vi "Errorbar1000.vi"   [LabVIEW 2013]
uses:
  <vilib>/Heliosphere Research LLC/Advanced Plotting Toolkit/Advanced Plotting Toolkit.lvlib
types:
  T1 = typedef "Advanced Plotting Toolkit.lvlib/PlotID.ctl" = i32
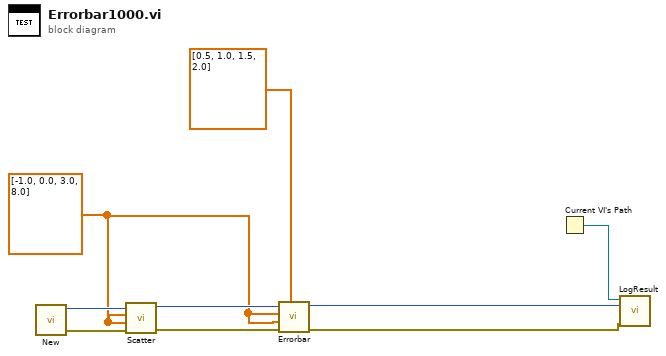
[diagram p0: block diagram]
diagram:
  w2 = dbl[] [-1.0, 0.0, 3.0, 8.0] ("X Data")
  n1 = call <vilib>:"New.vi"() -> ("error out"=w3:errorcluster, "Plot ID"=w6:T1)  [unwired: 10 in]
  n2 = call <vilib>:"Scatter.vi"("error in (no error)"=w3, "Y Data"=w2, "X Data"=w2, "Plot ID"=w6) -> ("error out"=w4:errorcluster, "Plot ID Out"=w5:T1)  [unwired: 6 in]
  n3 = call <vilib>:"Errorbar.vi"("X Errors"=dbl[] [0.5, 1.0, 1.5, 2.0], "error in (no error)"=w4, "Y Data"=w2, "X Data"=w2, "Plot ID"=w5) -> ("error out"=w7:errorcluster, "Plot ID out"=w8:T1)  [unwired: 5 in]
  n4 = Current VI's Path() -> (path=w9:path)
  n5 = call "LogResult.vi"("Test Result"=w7, "Test Artifact"=w8, "VI Path"=w9) -> ()  [unwired: 9 in]
